vi "RT_Main.vi"() -> ()   [LabVIEW 2018]
uses:
  controls/Data To Save.ctl
  controls/Control RT Code.ctl
  controls/Trial Config Settings.ctl
  <vilib>/Platform/TimedLoop/XDataNode/timing_clust.ctl
  <vilib>/Platform/TimedLoop/XDataNode/nitl_modes.ctl
  <vilib>/Platform/TimedLoop/XDataNode/wakeup.ctl
  controls/Rig Config Settings.ctl
  <vilib>/FPGAPlugInAG/cRIO-9045/niLvFpga_Open_cRIO-9045.vi
  <vilib>/rvi/interface/common/dynamic/niFpgaDynamicAddResources.vi
  <vilib>/FPGAPlugInAG/Dynamic/niLvFpga_Run_Dynamic.vi
  Globals/Global - Configuration Options.vi
  <vilib>/FPGAPlugInAG/Dynamic/niLvFpga_Close_Dynamic.vi
  <vilib>/Platform/TimedLoop/XDataNode/XDataNode.xnode
  <vilib>/rvi/interface/nirviOpenFPGA/nirviOpenFPGA.xnode
  FPGA Bitfiles/UIUCWhiskerProje_FPGATarget_FPGABuild_ja8qmgOJlMY.lvbitx
  FPGA_Main.vi
  <vilib>/rvi/interface/nirviMethod/nirviMethod.xnode
  <vilib>/rvi/interface/nirviCloseFPGA/nirviCloseFPGA.xnode
  <vilib>/Platform/TimedLoop/XDataNode/XDNodeRunTimeDep.lvlib
  <vilib>/NI_Real-Time Target Support.lvlib
  <vilib>/FPGAPlugInAG/Dynamic/niLvFpga_Abort_Dynamic.vi
  <vilib>/FPGAPlugInAG/Dynamic/niLvFpga_Reset_Dynamic.vi
panel:
  out "Group Size for Randomization":i32
  out "Trial Running Graph Flag":bool
  out "Trial#":i16
  out "Super Trial Group on Test":string[](array[string])
  in  "Inter Group Counter":dbl
  out "Super Trial Groups":i32
  out "Super Trial Groups":string[][](array[string])
  out "Start Test":bool
  out "Test Trial Plot Color Array":u32[](array[numeric])
  out "Test Trial Array":string[](array[string])
  out "Numeric":i32
  out "Flag - Lat Dist History":bool
  out "Lateral Trial History":dbl[][](array[numeric])
  out "# water at start of new trial":i32
  out "Array":T1[](array[typedef])
  out "RT Loop Finished Late?":bool
  out "cur_trial_distance":dbl
  out "Analog Inputs":sgl[](array[numeric])
  out "Analog Outputs":sgl[](array[numeric])
  out "DIO":bool[](array[boolean])
  out "Trial In Progress":T2
  out "Time into Trial":dbl
  out "Trial Config Index":i32
  in  "Inter-Trial Interval":bool
  out "Test Trial In Progress":string
  out "Trial Tracker":string[][](table)=[["Test Reward.dat", "9", "8"], ["Test NO Reward.dat", "8", "0"]]
  out "Array of Trial File Names":string[](array[string])
  in  "Test Trial Index":i32
  out "Array of Trials":T2[](array[typedef])
  out "Timeout Timer":dbl format="%.3f"
  out "Timeout?":bool
  out "Timeout SP":dbl caption="Timeout" format="%.1f"
  out "Trial Fraction":dbl format="%.2f"
  in  "Command RT Code":T1
  out "# elements":u32
  out "Flash Drive Directory":path=path "u:/"
  out "# of CPUs":u32
  out "Error Out":errorcluster
  in  "Error In":errorcluster
  out "Data To Save":T3 {"Seconds Into Trial(s)" format="%#.10g"}
  out "Trial Running":bool
  out "Loop Rate for High Priority Acq Loop":u32
  out "cRIO System Time":string
  out "cRIO System Date":string
  out "cRIO CPU1 Usage":dbl format="%.2f"
  out "cRIO CPU2 Usage":dbl format="%.2f"
  # "Inputs and Outputs"
  # "aClck_DI"
  # "frame_clock_DO"
  # "whisker_video_ctrl_DO"
  # "lick_signal_DO"
  # "water_valve_ctrl_DO"
  # "laser_ctrl"
  # "left_texture_ctrl_DO"
  # "right_texture_ctrl_DO"
  # "trial_ephys_ctrl_DO"
  # "trial_iti_ctrl_DO"
  # "trial_on_ctrl_DO"
  # "ephys_clock_DO"
  # "Timeout"
  # "cm"
  # "secs"
  # "secs"
  # "secs"
  # "msec"
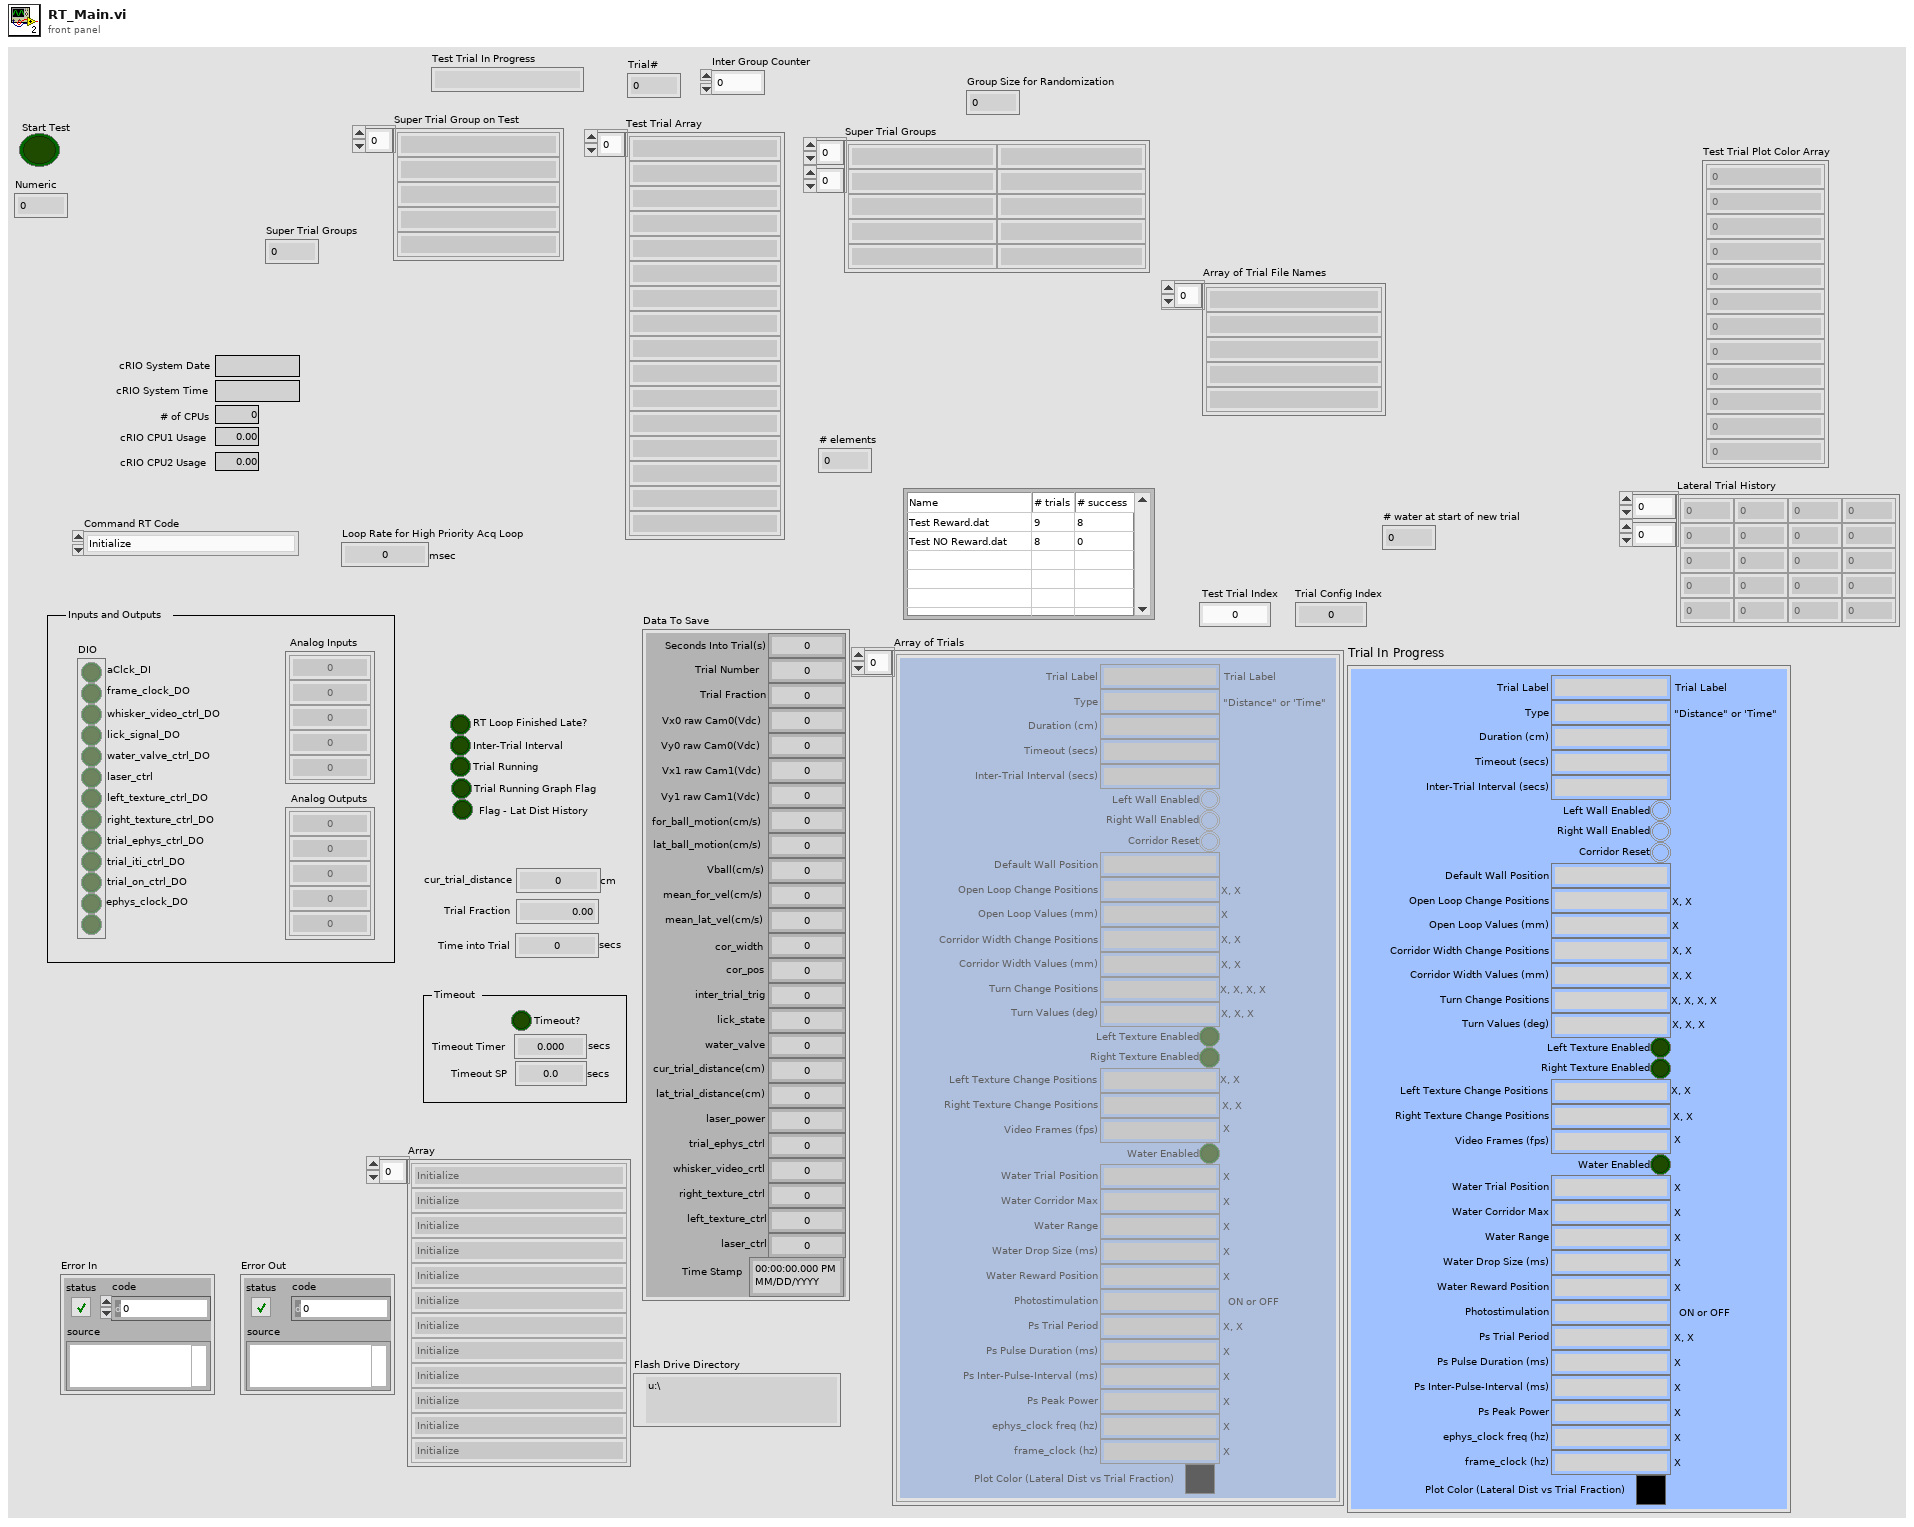
[diagram p1: front panel]
types:
  T1 = typedef "Control RT Code.ctl" = enum16{"Initialize", "Start New Test", "Stop Trial", "Start New Trial", "Load Trial Config Settings", "Load Rig Config Settings", "Determine Which Trial to Run", "Download All Trials to RT System", "Create New Folder", "Create New Data File", "Inter-Trial Interval Delay", "Initialize Trial Tracker", "Update Water Tracker", "Update Trial Tracker", "Exit"}
  T2 = typedef "Trial Config Settings.ctl" = cluster{"Trial Label":string, "Type":string, "Timeout (secs)":string, "Inter-Trial Interval (secs)":string, "Left Wall Enabled":bool, "Right Wall Enabled":bool, "Corridor Reset":bool, "Default Wall Position":string, "Open Loop Change Positions":string, "Open Loop Values (mm)":string, "Corridor Width Change Positions":string, "Corridor Width Values (mm) ":string, "Turn Change Positions":string, "Turn Values (deg)":string, "Left Texture Change Positions":string, "Right Texture Change Positions":string, "Video Frames (fps)":string, "Water Enabled":bool, "Water Trial Position":string, "Photostimulation":string, "Water Corridor Max":string, "Water Range":string, "Water Drop Size (ms)":string, "Water Reward Position":string, "Duration (cm)":string, "Left Texture Enabled":bool, "Right Texture Enabled":bool, "Ps Trial Period":string, "Ps Inter-Pulse-Interval (ms)":string, "Ps Peak Power":string, "Ps Pulse Duration (ms)":string, "ephys_clock freq (hz)":string, "frame_clock (hz)":string, "Plot Color (Lateral Dist vs Trial Fraction)":u32}
  T3 = typedef "Data To Save.ctl" = cluster{"Vx0 raw Cam0(Vdc)":sgl, "Vy0 raw Cam0(Vdc)":sgl, "Vx1 raw Cam1(Vdc)":sgl, "Vy1 raw Cam1(Vdc)":sgl, "Seconds Into Trial(s)":dbl, "cor_width":sgl, "cor_pos":sgl, "for_ball_motion(cm/s)":sgl, "lat_ball_motion(cm/s)":sgl, "Vball(cm/s)":sgl, "mean_for_vel(cm/s)":sgl, "mean_lat_vel(cm/s)":sgl, "Trial Fraction":dbl, "Trial Number":i16, "inter_trial_trig":i16, "lick_state":i16, "water_valve":i16, "cur_trial_distance(cm)":dbl, "lat_trial_distance(cm)":dbl, "laser_power":dbl, "trial_ephys_ctrl":i16, "whisker_video_crtl":i16, "right_texture_ctrl":i16, "left_texture_ctrl":i16, "laser_ctrl":i16, "Time Stamp":timestamp}
  T4 = cluster{"read mode":enum16{"polling", "blocking"}, "write mode":enum16{"polling", "blocking"}}
  T5 = enum16{"Create Folder", "Save", "Create New Data File"}
  T6 = typedef "XDNodeRunTimeDep.lvlib/timing_clust.ctl" = cluster{"Expected End [f-1]":u64, "Actual End [f-1]":u64, "Finished Late? [f-1]":bool, "Expected End [i-1]":u64, "Actual End [i-1]":u64, "Finished Late? [i-1]":bool, "Expected Start [i]":u64, "Actual Start [i]":u64, "Expected Start [f]":u64, "Actual Start [f]":u64, "Source Name":string, "Structure Name":string, "Period":i64, "Deadline":i64, "Offset":i64, "Start":i64, "Priority":i32, "Timeout":i32, "Mode":T7, "Wakeup Reason":T8, "Error":errorcluster, "Source Type":string, "Secondary Source Type":string, "Global End Time":u64, "Global Start Time":u64, "Frame Duration":u64, "Iteration Duration":u64, "Assigned CPU":i32, "I/O Scan Engine Mode":u32}
  T7 = typedef "XDNodeRunTimeDep.lvlib/nitl_modes.ctl" = enum32{"No Change", "Process missed periods, maintain original phase", "Discard missed periods, maintain original phase", "Process missed periods, ignore original phase", "Discard missed periods, ignore original phase"}
  T8 = typedef "XDNodeRunTimeDep.lvlib/wakeup.ctl" = enum32{"Normal", "Aborted", "Asynchronous wakeup", "Timing source error", "Timed loop error", "Timeout"}
  T9 = typedef "Rig Config Settings.ctl" = cluster{"Rig Name":string, "Rig Room":string, "Base Directory":string, "Computer IP Address":string, "Globals Name":string, "Treatmill Str":string, "cRIO Test Data Dir":path, "ai":string, "ao":string, "dio":string, "A_calib_str_row1":string, "A_calib_str_row2":string, "A_calib_str_row3":string, "Zero_V_str":string, "step_V":string, "Sample Freq":string, "ai_threshold":string, "run_speed_thresh":string, "speed_time_length":string, "wall ball gain":string, "max wall pos":string, "max cor width":string, "Trial Config Directory":path, "Randomize Trials?":bool}
  T10 = typedef "NI_Real-Time Target Support.lvlib/RT CPU Load.ctl" = cluster{"Total (%)":dbl, "Time Critical (%)":dbl, "Timed Structures (%)":dbl, "High (%)":dbl, "Above Normal (%)":dbl, "Normal (%)":dbl, "Background (%)":dbl, "Idle (%)":dbl, "ISR (%)":dbl}
  T11 = cluster{"Frequency (periods/tick)":fxp<+,32,0>, "Phase offset (periods)":fxp<+,32,0>, "Scale factor":fxp<+/-,16,1>, "Amplitude offset":fxp<+/-,16,16>, "duty cycle (periods)":fxp<+,32,0>}
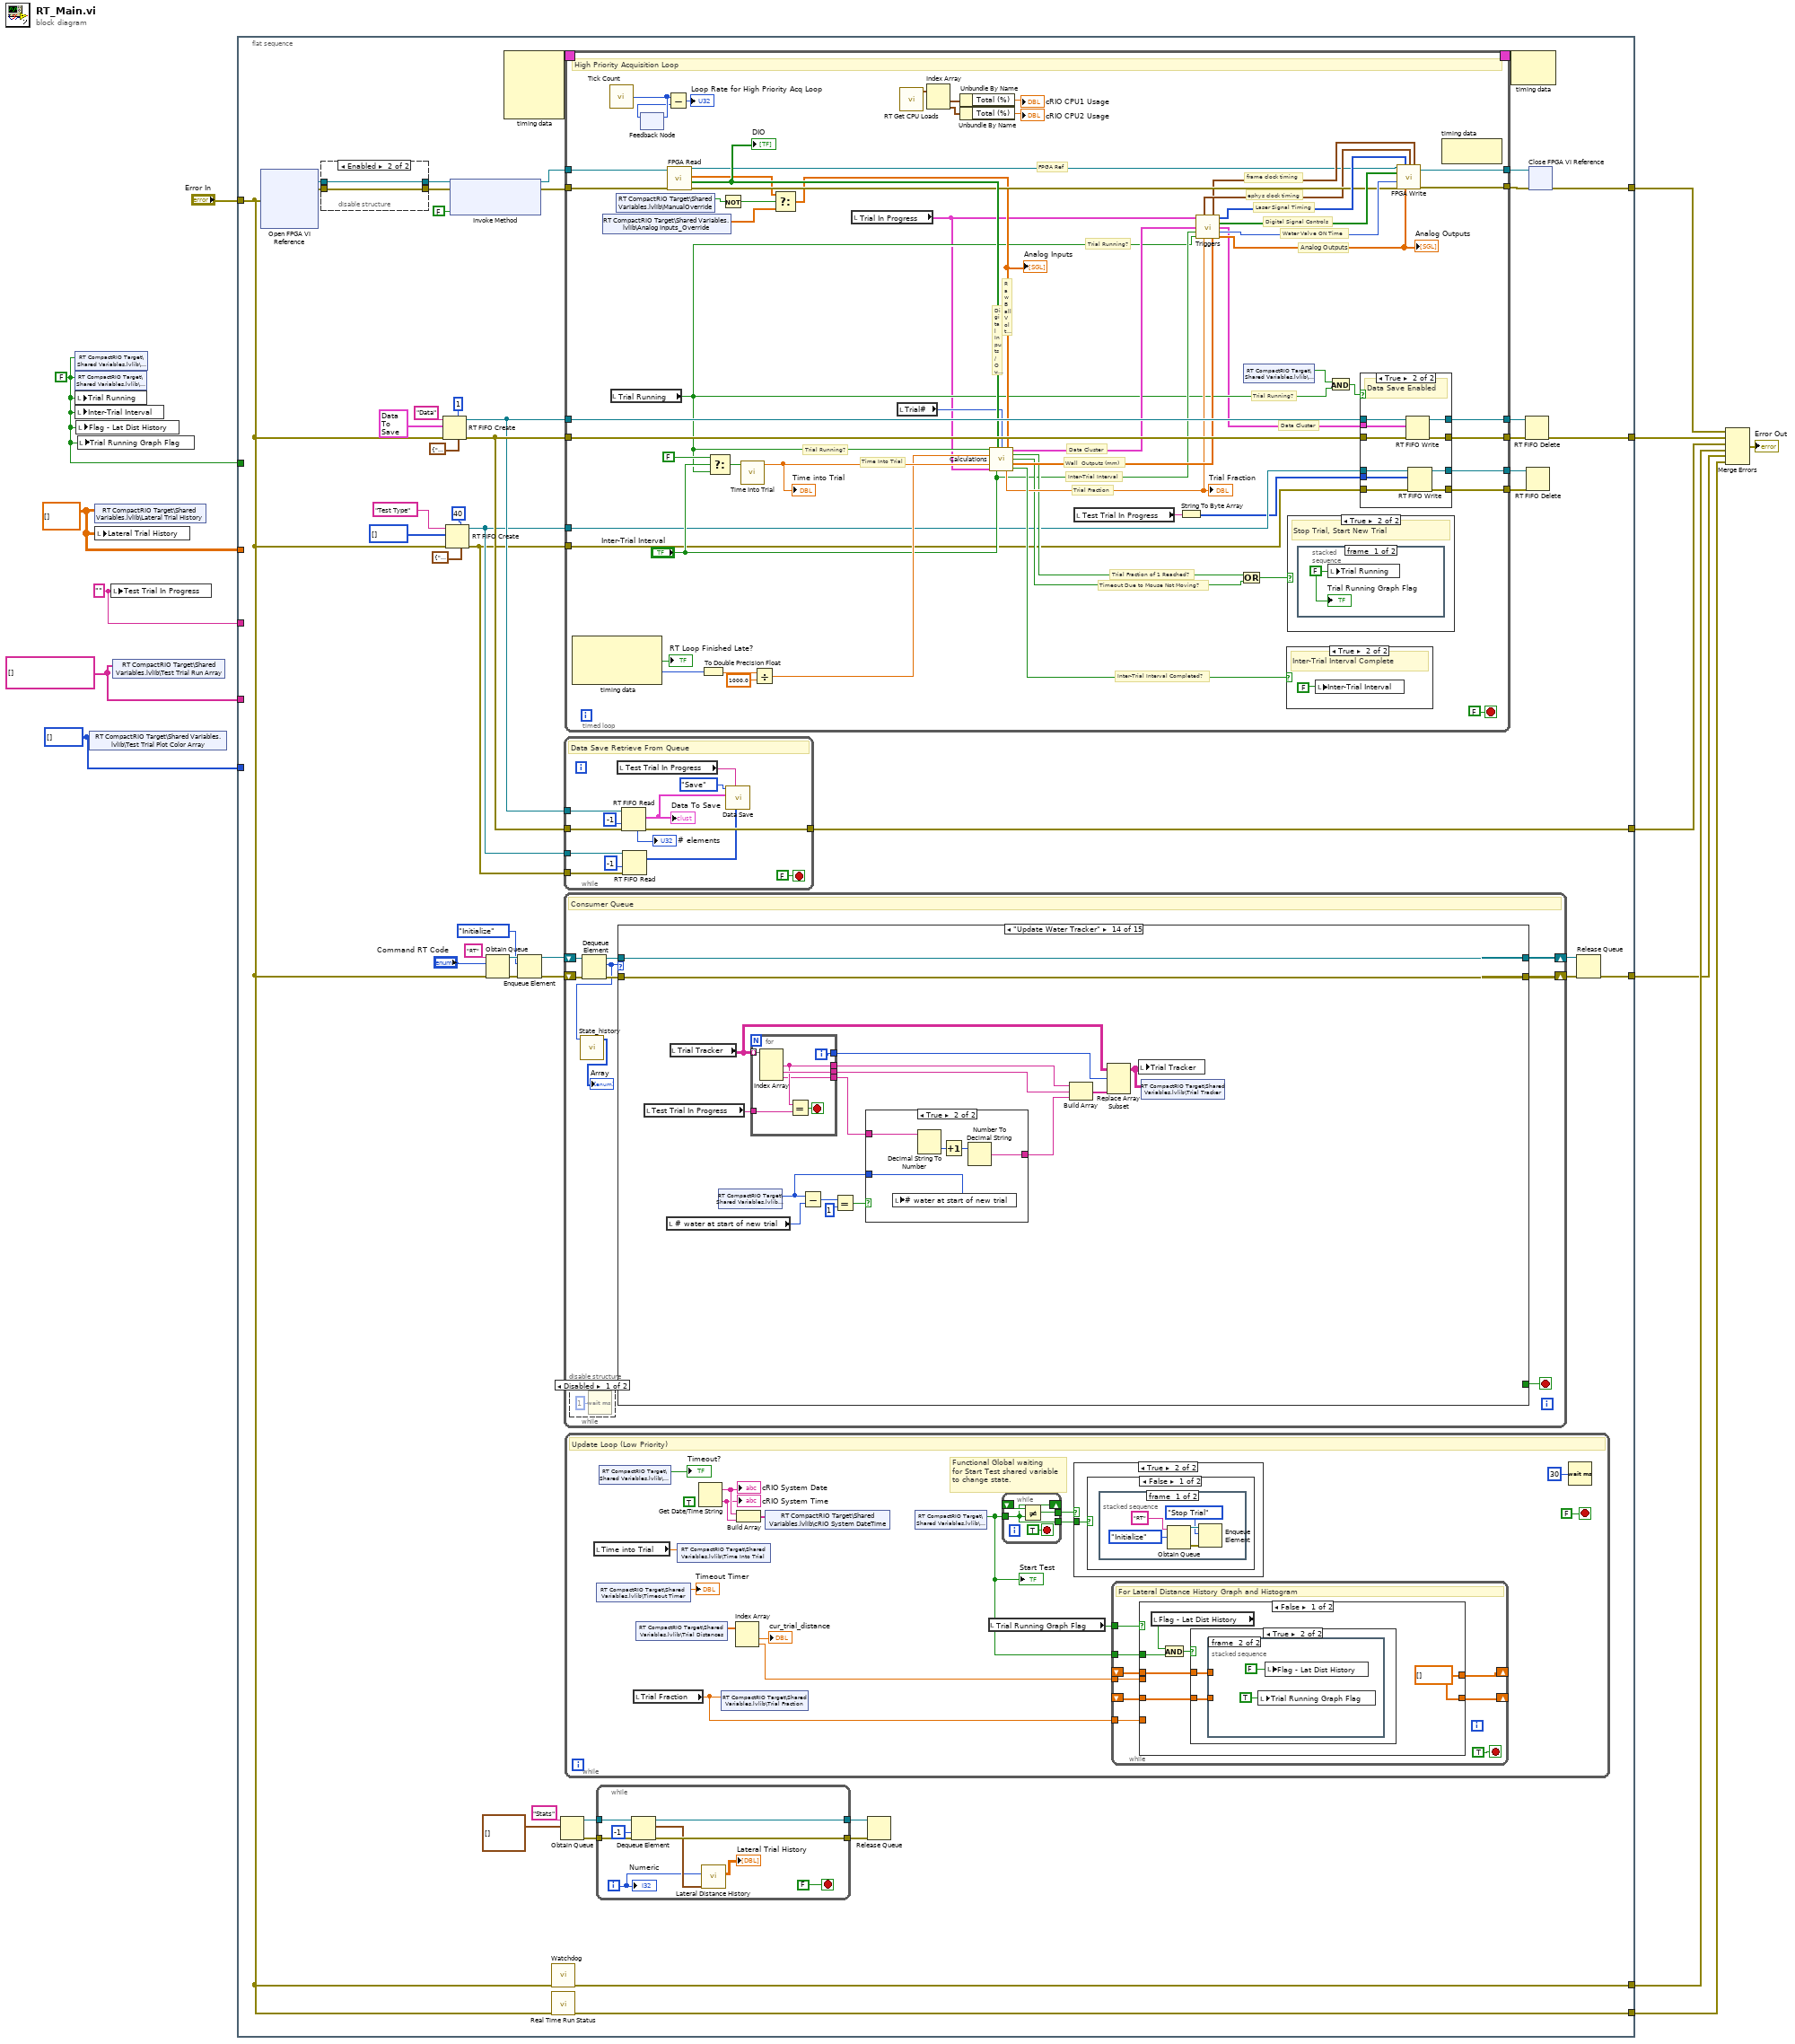
[diagram p0: block diagram]
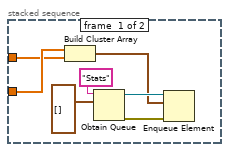
[diagram p3: hidden frame]
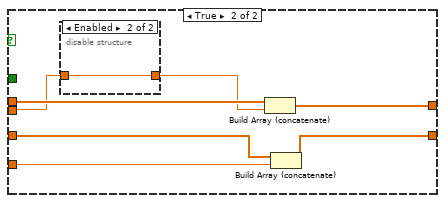
[diagram p4: hidden frame]
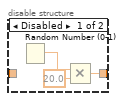
[diagram p5: hidden frame]
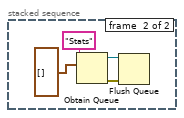
[diagram p7: hidden frame]
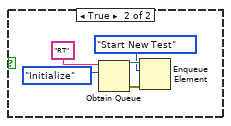
[diagram p8: hidden frame]
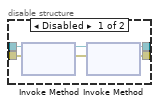
[diagram p9: hidden frame]
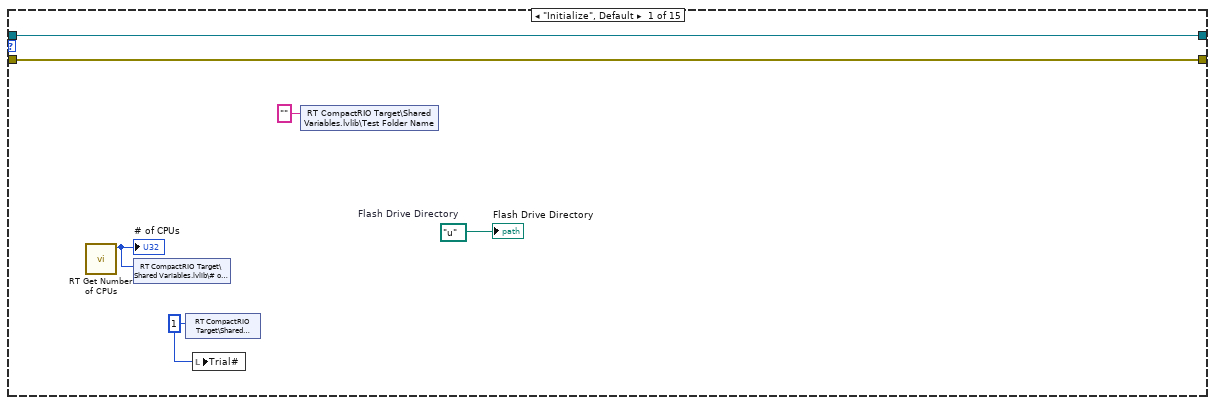
[diagram p11: hidden frame]
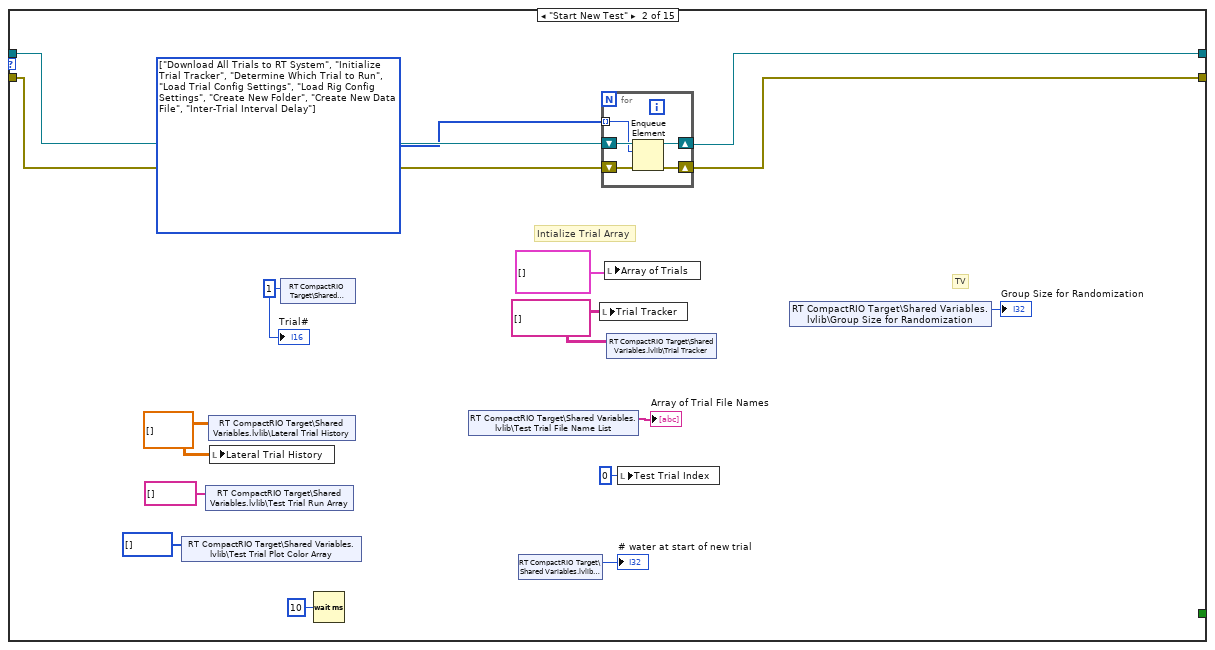
[diagram p12: hidden frame]
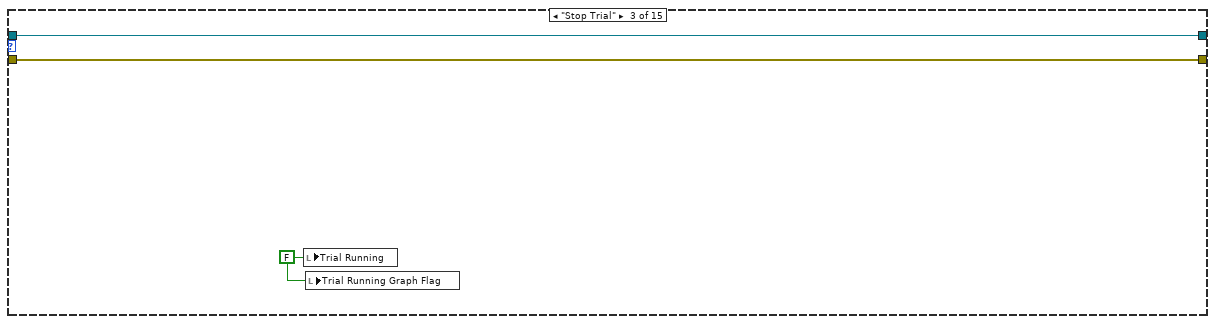
[diagram p13: hidden frame]
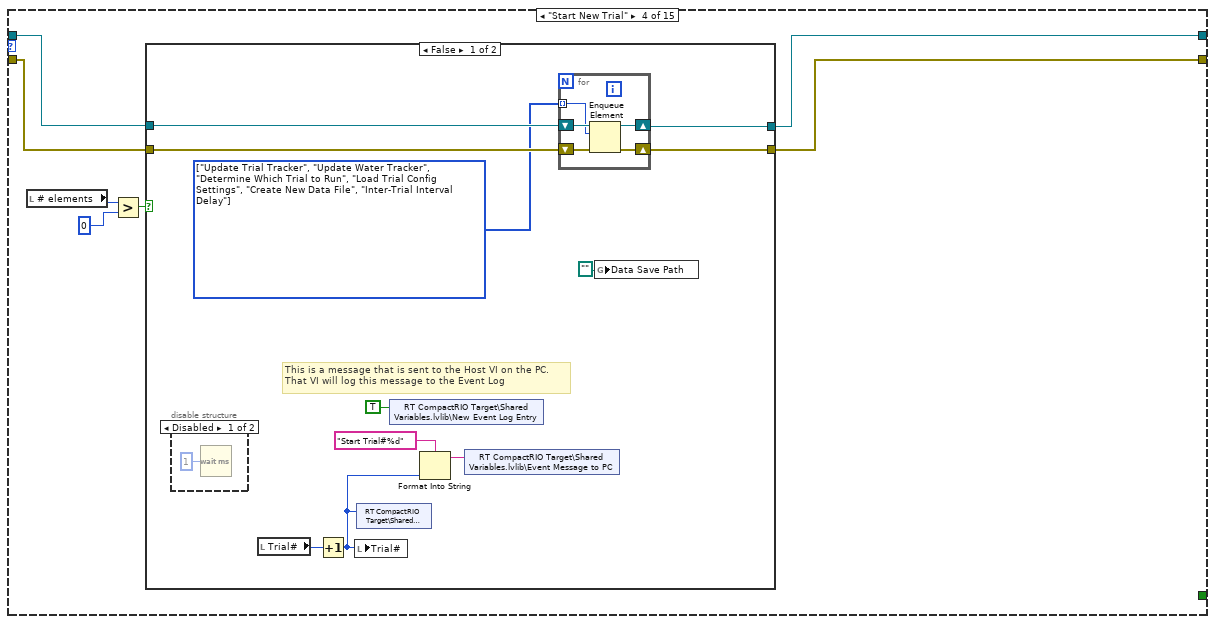
[diagram p14: hidden frame]
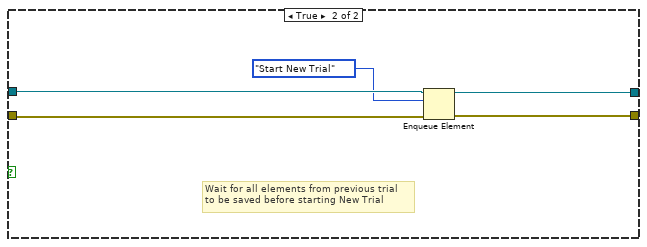
[diagram p16: hidden frame]
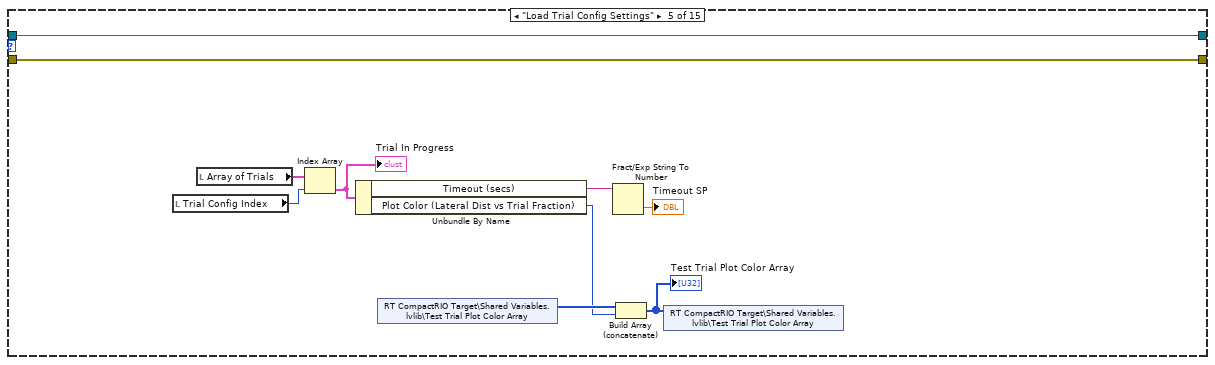
[diagram p17: hidden frame]
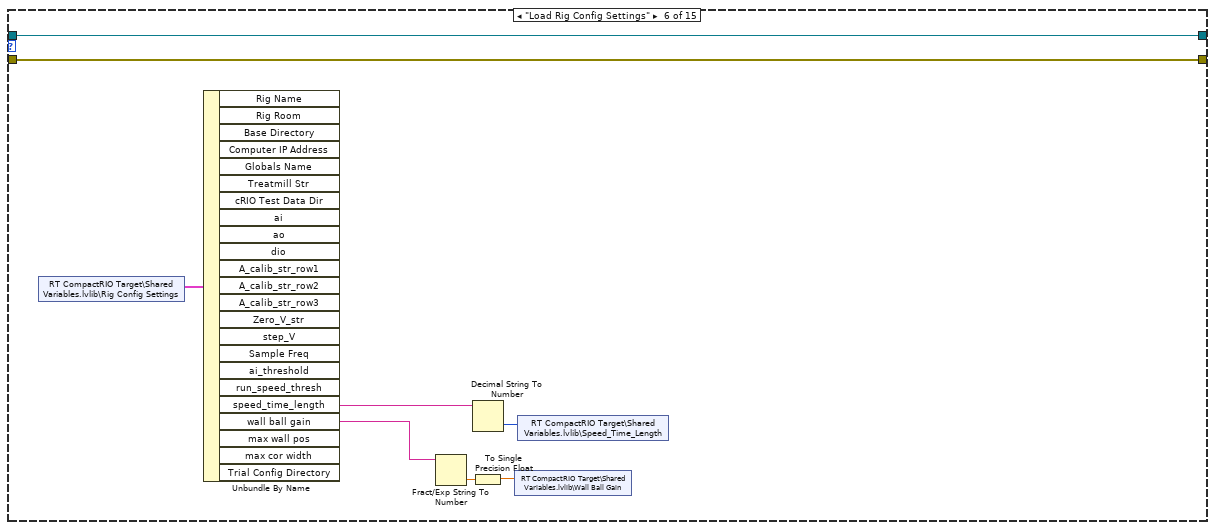
[diagram p18: hidden frame]
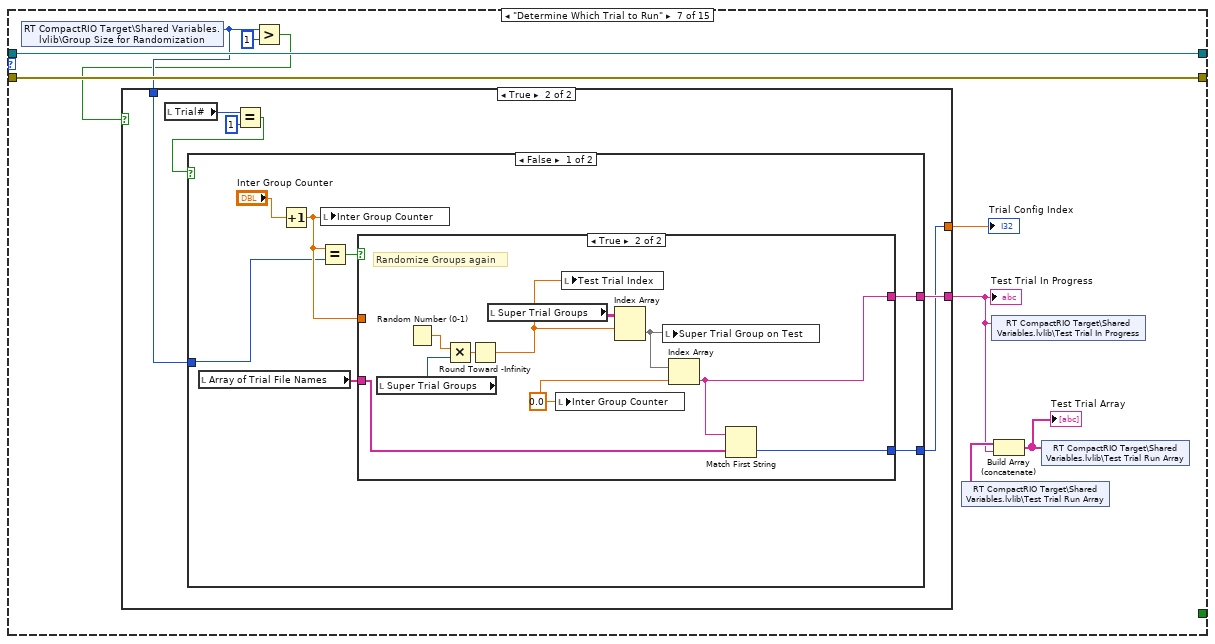
[diagram p19: hidden frame]
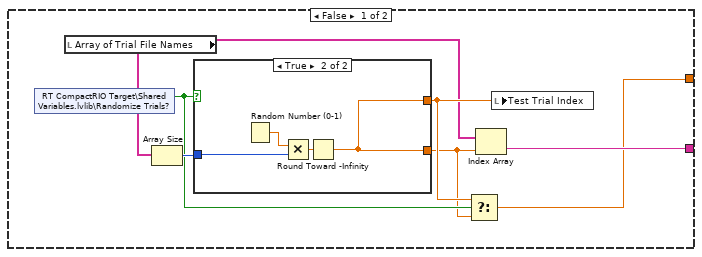
[diagram p20: hidden frame]
diagram:
  w2 = u32[] [] ("Test Trial Plot Color Array")
  w3 = string[] [] ("Test Trial Run Array")
  w4 = "" ("Test Trial In Progress")
  w5 = dbl[][] [] ("Histogram Data")
  w1 = FALSE ("Start Test for FPGA")
  n1 = shared-variable "RT CompactRIO Target\\Shared Variables.lvlib\\Timeout?"(w1) -> ()  [unwired: 1 in, 1 out]
  n2 = shared-variable "RT CompactRIO Target\\Shared Variables.lvlib\\Start Test"(w1) -> ()  [unwired: 1 in, 1 out]
  n3 = local write "Trial Running"(w1) -> ()
  n4 = local write "Inter-Trial Interval"(w1) -> ()
  n5 = local write "Flag - Lat Dist History"(w1) -> ()
  n6 = local write "Trial Running Graph Flag"(w1) -> ()
  n7 = shared-variable "RT CompactRIO Target\\Shared Variables.lvlib\\Test Trial Plot Color Array"(w2) -> ()  [unwired: 1 in, 1 out]
  n8 = shared-variable "RT CompactRIO Target\\Shared Variables.lvlib\\Lateral Trial History"(w5) -> ()  [unwired: 1 in, 1 out]
  n9 = local write "Lateral Trial History"(w5) -> ()
  n10 = local write "Test Trial In Progress"(w4) -> ()
  n11 = shared-variable "RT CompactRIO Target\\Shared Variables.lvlib\\Test Trial Run Array"(w3) -> ()  [unwired: 1 in, 1 out]
  n12 = flat-sequence {
    tunnel: [w54] -> w13
    tunnel: [w50] -> w12
    tunnel: [w44] -> w11
    tunnel: [w53] -> w10
    tunnel: [w47] -> w8
    tunnel: [w31] -> w7
    tunnel: "Error In" -> [w18]
    tunnel: w1 -> [_]
    tunnel: w5 -> [_]
    tunnel: w4 -> [_]
    tunnel: w3 -> [_]
    tunnel: w2 -> [_]
    frame #0 {
      n13 = xnode "Open FPGA VI Reference"("error in"=w18) -> ("FPGA VI Reference Out"=w48:refnum<k20>, "error out"=w57:errorcluster)  [unwired: 1 in]
      n14 = disable-structure shown="Enabled" {
        disable-tunnel: [w162 w164] -> w58
        disable-tunnel: w48 -> [w160 w164]
        disable-tunnel: w57 -> [w159 w163]
        disable-tunnel: [w157 w163] -> w56
        frame Disabled {
          n15 = xnode "Invoke Method"("FPGA VI Reference In"=w160, "error in"=w159) -> ("FPGA VI Reference Out"=w161:refnum<k20>, "error out"=w158:errorcluster)
          n16 = xnode "Invoke Method"("FPGA VI Reference In"=w161, "error in"=w158) -> ("FPGA VI Reference Out"=w162:refnum<k20>, "error out"=w157:errorcluster)
        }
        frame Enabled {
        }
      }
      n17 = RT FIFO Create(0:"Data" ("name (unnamed)"), 1:T3 {"Vx0 raw Cam0(Vdc)"=0.0, "Vy0 raw Cam0(Vdc)"=0.0, "Vx1 raw Cam1(Vdc)"=0.0, "Vy1 raw Cam1(Vdc)"=0.0, "Seconds Into Trial(s)"=0.0, "cor_width"=0.0, "cor_pos"=0.0, "for_ball_motion(cm/s)"=0.0, "lat_ball_motion(cm/s)"=0.0, "Vball(cm/s)"=0.0, "mean_for_vel(cm/s)"=0.0, "mean_lat_vel(cm/s)"=0.0, "Trial Fraction"=0.0, "Trial Number"=0, "inter_trial_trig"=0, "lick_state"=0, "water_valve"=0, "cur_trial_distance(cm)"=0.0, "lat_trial_distance(cm)"=0.0, "laser_power"=0.0, "trial_ephys_ctrl"=0, "whisker_video_crtl"=0, "right_texture_ctrl"=0, "left_texture_ctrl"=0, "laser_ctrl"=0, "Time Stamp"=timestamp(0 s since 1904-01-01)} ("Data Cluster OUT"), 3:w18, 6:u32 1 ("elements in array (1)"), 7:T4 {"read mode"=enum."blocking", "write mode"=enum."blocking"} ("r/w modes (polling,polling)")) -> (8:w45:refnum<k33>, 11:w46:errorcluster)  [unwired: 3 in, 1 out]
      n18 = RT FIFO Create(0:"Test Type" ("name (unnamed)"), 1:u8[] [] ("Trial Type"), 3:w18, 6:u32 40 ("elements in array (1)"), 7:T4 {"read mode"=enum."blocking", "write mode"=enum."blocking"} ("r/w modes (polling,polling)")) -> (8:w17:refnum<k33>, 11:w15:errorcluster)  [unwired: 3 in, 1 out]
      n19 = xnode "Invoke Method"("FPGA VI Reference In"=w58, "error in"=w56, "Wait Until Done (F)"=FALSE) -> ("FPGA VI Reference Out"=w49:refnum<k20>, "error out"=w59:errorcluster)
      n20 = Obtain Queue(name (unnamed)="RT", element data type="Command RT Code", error in (no error)=w18) -> (queue out=w40:refnum<queue>, error out=w41:errorcluster)  [unwired: 2 in, 1 out]
      n21 = node-c288() -> (w62:T6)  [unwired: 4 in]
      n22 = Enqueue Element(queue=w40, element=Control_RT_Code."Initialize", error in (no error)=w41) -> (queue out=w38:refnum<queue>, error out=w37:errorcluster)  [unwired: 1 in, 1 out]
      n23 = call "Watchdog.vi"("Error IN"=w18) -> ("Error Out"=w53:errorcluster)  [unwired: 10 in]
      n24 = call "Real Time Run Status.vi"("Error IN"=w18) -> ("Error OUT"=w47:errorcluster)  [unwired: 9 in, 1 out]
      n25 = Obtain Queue(name (unnamed)="Stats", element data type=cluster{"Numeric":dbl, "Numeric":dbl}[] [] ("array of clusters")) -> (queue out=w26:refnum<queue>, error out=w25:errorcluster)  [unwired: 3 in, 1 out]
      n26 = while {
        tunnel: [w156] -> w44
        tunnel: w46 -> [w155]
        tunnel: w45 -> [w154]
        tunnel: w15 -> [w146]
        tunnel: w17 -> [w145]
        stop <- FALSE stop-if-true
        # "Data Save Retrieve From Queue"
        n27 = local read "Test Trial In Progress"() -> (w149:string)
        n28 = RT FIFO Read(0:w154, 2:-1 ("timeout in ms (0)"), 3:w155) -> (7:→"# elements":u32, 9:w148:T3, 11:w156:errorcluster)  [unwired: 1 in, 2 out]
        "Data To Save" <- w148
        n29 = RT FIFO Read(0:w145, 2:-1 ("timeout in ms (0)"), 3:w146) -> (9:w144:u8[])  [unwired: 1 in, 4 out]
        n30 = call "Data Save.vi"("Test Type"=w144, "Test Trial In Progress"=w149, "Data Cluster"=w148, "Task"=T5."Save") -> ()  [unwired: 6 in, 2 out]
      }
      n31 = while {
        shift-right: [w169] -> w34
        shift-left: w38 -> [w173]
        shift-right: [w168] -> w33
        shift-left: w37 -> [w172]
        stop <- w167 stop-if-true
        # "Consumer Queue"
        n32 = disable-structure shown="Disabled" {
          frame Disabled {
            n33 = Wait (ms)(milliseconds to wait=u32 1) -> ()  [unwired: 1 out]
          }
          frame Enabled {
          }
        }
        n34 = Dequeue Element(queue=w173, error in (no error)=w172) -> (queue out=w171:refnum<queue>, element=w166:T1, error out=w170:errorcluster)  [unwired: 1 in, 1 out]
        n35 = call "State_history.vi"("element"=w166) -> ("Array"=→"Array":T1[])  [unwired: 10 in]
        n36 = case shown="\"Update Water Tracker\"" w166 {
          tunnel: w171 -> [w178 w196 w204 w211 w243 w251 w260 w327 w331 w341 w368 w375 w399 w422 w438]
          tunnel: w170 -> [w177 w193 w203 w208 w238 w250 w259 w326 w330 w340 w367 w374 w398 w421 w437]
          tunnel: [w178 w195 w204 w210 w243 w251 w260 w327 w331 w341 w368 w375 w399 w422 w438] -> w169
          tunnel: [w177 w194 w203 w209 w238 w250 w259 w326 w329 w339 w367 w374 w398 w421 w437] -> w168
          tunnel: [_ _ _ _ _ _ _ _ _ _ _ _ _ _ TRUE] -> w167
          frame "Initialize", Default {
            w175 = 1 ("Trial#")
            w179 = path "u:/"  # Flash Drive Directory
            n37 = call <vilib>:"RT Get Number of CPUs.vi"() -> ("# of CPUs"=w180:u32)  [unwired: 10 in, 1 out]
            "# of CPUs" <- w180
            n38 = shared-variable "RT CompactRIO Target\\Shared Variables.lvlib\\# of CPUs"(w180) -> ()  [unwired: 1 in, 1 out]
            n39 = shared-variable "RT CompactRIO Target\\Shared Variables.lvlib\\Trial#"(w175) -> ()  [unwired: 1 in, 1 out]
            n40 = local write "Trial#"(w175) -> ()
            n41 = shared-variable "RT CompactRIO Target\\Shared Variables.lvlib\\Test Folder Name"("" ("Test Folder Name")) -> ()  [unwired: 1 in, 1 out]
            "Flash Drive Directory" <- w179
          }
          frame "Start New Test" {
            w183 = 1 ("Trial#")
            w187 = dbl[][] [] ("Histogram Data")
            w186 = string[][] [] ("Trial Tracker")
            w192 = T1[] [enum."Download All Trials to RT System", enum."Initialize Trial Tracker", enum."Determine Which Trial to Run", enum."Load Trial Config Settings", enum."Load Rig Config Settings", enum."Create New Folder", enum."Create New Data File", enum."Inter-Trial Interval Delay"] items=["Initialize", "Start New Test", "Stop Trial", "Start New Trial", "Load Trial Config Settings", "Load Rig Config Settings", "Determine Which Trial to Run", "Download All Trials to RT System", "Create New Folder", "Create New Data File", "Inter-Trial Interval Delay", "Initialize Trial Tracker", "Update Water Tracker", "Update Trial Tracker", "Exit"]
            # "TV"
            # "Intialize Trial Array"
            n42 = shared-variable "RT CompactRIO Target\\Shared Variables.lvlib\\Test Trial Plot Color Array"(u32[] [] ("Test Trial Plot Color Array")) -> ()  [unwired: 1 in, 1 out]
            n43 = shared-variable "RT CompactRIO Target\\Shared Variables.lvlib\\Test Trial Run Array"(string[] [] ("Test Trial Run Array")) -> ()  [unwired: 1 in, 1 out]
            n44 = shared-variable "RT CompactRIO Target\\Shared Variables.lvlib\\Lateral Trial History"(w187) -> ()  [unwired: 1 in, 1 out]
            n45 = local write "Lateral Trial History"(w187) -> ()
            n46 = shared-variable "RT CompactRIO Target\\Shared Variables.lvlib\\Trial#"(w183) -> ()  [unwired: 1 in, 1 out]
            n47 = Wait (ms)(milliseconds to wait=u32 10) -> ()  [unwired: 1 out]
            n48 = shared-variable "RT CompactRIO Target\\Shared Variables.lvlib\\Test Trial File Name List"() -> (→"Array of Trial File Names":string[])  [unwired: 1 in, 1 out]
            n49 = shared-variable "RT CompactRIO Target\\Shared Variables.lvlib\\# water"() -> (→"# water at start of new trial":i32)  [unwired: 1 in, 1 out]
            n50 = local write "Trial Tracker"(w186) -> ()
            n51 = for {
              shift-right: [w200] -> w195
              shift-left: w196 -> [w201]
              shift-right: [w198] -> w194
              shift-left: w193 -> [w199]
              tunnel: w192 -> [w197] mode=indexing
              n52 = Enqueue Element(queue=w201, element=w197, error in (no error)=w199) -> (queue out=w200:refnum<queue>, error out=w198:errorcluster)  [unwired: 1 in, 1 out]
            }
            n53 = local write "Array of Trials"(T2[] [] ("Array")) -> ()
            n54 = shared-variable "RT CompactRIO Target\\Shared Variables.lvlib\\Trial Tracker"(w186) -> ()  [unwired: 1 in, 1 out]
            n55 = local write "Test Trial Index"(0 ("Test Trial Index")) -> ()
            n56 = shared-variable "RT CompactRIO Target\\Shared Variables.lvlib\\Group Size for Randomization"() -> (→"Group Size for Randomization":i32)  [unwired: 1 in, 1 out]
            "Trial#" <- w183
          }
          frame "Stop Trial" {
            w202 = FALSE ("Trial Running")
            n57 = local write "Trial Running"(w202) -> ()
            n58 = local write "Trial Running Graph Flag"(w202) -> ()
          }
          frame "Start New Trial" {
            n59 = local read "# elements"() -> (w207:u32)
            n60 = Greater?(x=w207, y=u32 0) -> (0:w205:bool)
            n61 = case shown="False" w205 {
              tunnel: w211 -> [w222 w231]
              tunnel: [w221 w233] -> w210
              tunnel: [w220 w232] -> w209
              tunnel: w208 -> [w219 w230]
              frame False {
                w218 = T1[] [enum."Update Trial Tracker", enum."Update Water Tracker", enum."Determine Which Trial to Run", enum."Load Trial Config Settings", enum."Create New Data File", enum."Inter-Trial Interval Delay"] items=["Initialize", "Start New Test", "Stop Trial", "Start New Trial", "Load Trial Config Settings", "Load Rig Config Settings", "Determine Which Trial to Run", "Download All Trials to RT System", "Create New Folder", "Create New Data File", "Inter-Trial Interval Delay", "Initialize Trial Tracker", "Update Water Tracker", "Update Trial Tracker", "Exit"]
                # "This is a message that is sent to the Host VI on the PC.\nThat VI will log this message to the Event Log"
                n62 = disable-structure shown="Disabled" {
                  frame Disabled {
                    n63 = Wait (ms)(milliseconds to wait=u32 1) -> ()  [unwired: 1 out]
                  }
                  frame Enabled {
                  }
                }
                n64 = local read "Trial#"() -> (w213:i16)
                n65 = Increment(x=w213) -> (x+1=w212:i16)
                n66 = local write "Trial#"(w212) -> ()
                n67 = shared-variable "RT CompactRIO Target\\Shared Variables.lvlib\\Trial#"(w212) -> ()  [unwired: 1 in, 1 out]
                n68 = shared-variable "RT CompactRIO Target\\Shared Variables.lvlib\\New Event Log Entry"(TRUE ("New Event Log Entry")) -> ()  [unwired: 1 in, 1 out]
                n69 = Format Into String(format string="Start Trial#%d", w212) -> (resulting string=w214:string)  [unwired: 2 in, 1 out]
                n70 = shared-variable "RT CompactRIO Target\\Shared Variables.lvlib\\Event Message to PC"(w214) -> ()  [unwired: 1 in, 1 out]
                n71 = for {
                  shift-right: [w227] -> w221
                  shift-left: w222 -> [w228]
                  shift-right: [w225] -> w220
                  shift-left: w219 -> [w226]
                  tunnel: w218 -> [w224] mode=indexing
                  n72 = Enqueue Element(queue=w228, element=w224, error in (no error)=w226) -> (queue out=w227:refnum<queue>, error out=w225:errorcluster)  [unwired: 1 in, 1 out]
                }
                n73 = global write "Global - Configuration Options.vi" "Data Save Path"(path "") -> ()
              }
              frame True {
                # "Wait for all elements from previous trial\nto be saved before starting New Trial"
                n74 = Enqueue Element(queue=w231, element=Control_RT_Code."Start New Trial", error in (no error)=w230) -> (queue out=w233:refnum<queue>, error out=w232:errorcluster)  [unwired: 1 in, 1 out]
              }
            }
          }
          frame "Load Trial Config Settings" {
            n75 = local read "Trial Config Index"() -> (w237:i32)
            n76 = local read "Array of Trials"() -> (w240:T2[])
            n77 = Index Array(array=w240, index=w237) -> (element=w239:T2)
            "Trial In Progress" <- w239
            n78 = Unbundle By Name(w239) -> ("Timeout (secs)"=w241:string, "Plot Color (Lateral Dist vs Trial Fraction)"=w235:u32)
            n79 = shared-variable "RT CompactRIO Target\\Shared Variables.lvlib\\Test Trial Plot Color Array"() -> (w236:u32[])  [unwired: 1 in, 1 out]
            n80 = Fract/Exp String To Number(string=w241) -> (number=→"Timeout SP":dbl)  [unwired: 3 in, 1 out]
            n81 = Build Array (concatenate)(w236, w235) -> (w234:u32[])
            "Test Trial Plot Color Array" <- w234
            n82 = shared-variable "RT CompactRIO Target\\Shared Variables.lvlib\\Test Trial Plot Color Array"(w234) -> ()  [unwired: 1 in, 1 out]
          }
          frame "Load Rig Config Settings" {
            n83 = shared-variable "RT CompactRIO Target\\Shared Variables.lvlib\\Rig Config Settings"() -> (w249:T9)  [unwired: 1 in, 1 out]
            n84 = Unbundle By Name(w249) -> ("speed_time_length"=w248:string, "wall ball gain"=w246:string)  [unwired: 21 out]
            n85 = Fract/Exp String To Number(string=w246) -> (number=w245:dbl)  [unwired: 3 in, 1 out]
            n86 = Decimal String To Number(string=w248) -> (number=w247:i32)  [unwired: 2 in, 1 out]
            n87 = To Single Precision Float(number=w245) -> (single precision float=w244:sgl)
            n88 = shared-variable "RT CompactRIO Target\\Shared Variables.lvlib\\Wall Ball Gain"(w244) -> ()  [unwired: 1 in, 1 out]
            n89 = shared-variable "RT CompactRIO Target\\Shared Variables.lvlib\\Speed_Time_Length"(w247) -> ()  [unwired: 1 in, 1 out]
          }
          frame "Determine Which Trial to Run" {
            n90 = shared-variable "RT CompactRIO Target\\Shared Variables.lvlib\\Group Size for Randomization"() -> (w254:i32)  [unwired: 1 in, 1 out]
            n91 = Greater?(x=w254, y=1) -> (0:w253:bool)
            n92 = case shown="True" w253 {
              tunnel: [w262 w284] -> w256
              tunnel: w254 -> [_ w283]
              tunnel: [w261 w280] -> w252
              frame False {
                n93 = shared-variable "RT CompactRIO Target\\Shared Variables.lvlib\\Randomize Trials?"() -> (w264:bool)  [unwired: 1 in, 1 out]
                n94 = local read "Array of Trial File Names"() -> (w266:string[])
                n95 = Array Size(array=w266) -> (size(s)=w265:i32)
                n96 = case shown="True" w264 {
                  tunnel: [w270 w275] -> w263
                  tunnel: w265 -> [w272 w276]
                  tunnel: [w269 w275] -> w267
                  frame False {
                    n97 = Decrement(x=w272) -> (x-1=w271:i32)
                    n98 = Greater?(x="Test Trial Index", y=w271) -> (0:w274:bool)
                    n99 = Select(t=0, s=w274, f="Test Trial Index") -> (s? t:f=w270:i32)
                    n100 = Increment(x=w270) -> (x+1=w269:i32)
                  }
                  frame True {
                    n101 = Random Number (0-1)() -> (number: 0 to 1=w278:dbl)
                    n102 = Multiply(x=w278, y=w276) -> (x*y=w277:dbl)
                    n103 = Round Toward -Infinity(1:w277) -> (0:w275:dbl)
                  }
                }
                n104 = Select(t=w267, s=w264, f=w263) -> (s? t:f=w261:dbl)
                n105 = Index Array(array=w266, index=w263) -> (element=w262:string)
                n106 = local write "Test Trial Index"(w267) -> ()
              }
              frame True {
                n107 = local read "Trial#"() -> (w279:i16)
                n108 = Equal?(x=w279, y=1) -> (x = y?=w281:bool)
                n109 = case shown="False" w281 {
                  tunnel: [w287 w309] -> w284
                  tunnel: w283 -> [w286 w308]
                  tunnel: [w285 w307] -> w280
                  frame False {
                    n110 = local read "Array of Trial File Names"() -> (w291:string[])
                    n111 = Increment(x="Inter Group Counter") -> (x+1=w290:dbl)
                    n112 = Equal?(x=w290, y=w286) -> (x = y?=w289:bool)
                    n113 = local write "Inter Group Counter"(w290) -> ()
                    n114 = case shown="True" w289 {
                      tunnel: w290 -> [w295 _]
                      tunnel: w291 -> [w294 w299]
                      tunnel: [w293 w298] -> w287
                      tunnel: [w292 w297] -> w285
                      frame False {
                        n115 = local read "Super Trial Group on Test"() -> (w296:string[])
                        n116 = Index Array(array=w296, index=w295) -> (element=w293:string)
                        n117 = Match First String(2:w294, 3:w293) -> (0:w292:i32)  [unwired: 1 out]
                      }
                      frame True {
                        w301 = 0.0 ("Inter Group Counter")
                        # "Randomize Groups again"
                        n118 = local read "Super Trial Groups"() -> (w304:i32)
                        n119 = Random Number (0-1)() -> (number: 0 to 1=w306:dbl)
                        n120 = Multiply(x=w306, y=w304) -> (x*y=w305:dbl)
                        n121 = Round Toward -Infinity(1:w305) -> (0:w300:dbl)
                        n122 = local read "Super Trial Groups"() -> (w303:string[][])
                        n123 = local write "Inter Group Counter"(w301) -> ()
                        n124 = local write "Test Trial Index"(w300) -> ()
                        n125 = Index Array(array=w303, index (row)=w300) -> (element=w302:string[])  [unwired: 1 in]
                        n126 = local write "Super Trial Group on Test"(w302) -> ()
                        n127 = Index Array(array=w302, index=w301) -> (element=w298:string)
                        n128 = Match First String(2:w299, 3:w298) -> (0:w297:i32)  [unwired: 1 out]
                      }
                    }
                  }
                  frame True {
                    w317 = 0.0 ("Inter Group Counter")
                    n129 = local read "Array of Trial File Names"() -> (w319:string[])
                    n130 = Array Size(array=w319) -> (size(s)=w311:i32)
                    n131 = Divide(x=w311, y=w308) -> (x/y=w314:dbl)
                    "Super Trial Groups" <- w314
                    n132 = for {
                      N: w314 -> [_]
                      tunnel: w319 -> [w324]
                      tunnel: w308 -> [w322]
                      shift-right: [w320] -> _
                      shift-left: 0 -> [w323]
                      tunnel: [w321] -> w315 mode=indexing
                      n133 = Add(x=w323, y=w322) -> (x+y=w320:i32)
                      n134 = Array Subset(array=w324, index=w323, length=w322) -> (w321:string[])
                    }
                    "Super Trial Groups" <- w315
                    n135 = Random Number (0-1)() -> (number: 0 to 1=w313:dbl)
                    n136 = Multiply(x=w313, y=w314) -> (x*y=w312:dbl)
                    n137 = Round Toward -Infinity(1:w312) -> (0:w318:dbl)
                    n138 = Index Array(array=w315, index (row)=w318) -> (element=w316:string[])  [unwired: 1 in]
                    "Super Trial Group on Test" <- w316
                    n139 = local write "Test Trial Index"(w318) -> ()
                    n140 = local write "Inter Group Counter"(w317) -> ()
                    n141 = Index Array(array=w316, index=w317) -> (element=w309:string)
                    n142 = Match First String(2:w319, 3:w309) -> (0:w307:i32)  [unwired: 1 out]
                  }
                }
              }
            }
            "Test Trial In Progress" <- w256
            "Trial Config Index" <- w252
            n143 = shared-variable "RT CompactRIO Target\\Shared Variables.lvlib\\Test Trial Run Array"() -> (w258:string[])  [unwired: 1 in, 1 out]
            n144 = shared-variable "RT CompactRIO Target\\Shared Variables.lvlib\\Test Trial In Progress"(w256) -> ()  [unwired: 1 in, 1 out]
            n145 = Build Array (concatenate)(w258, w256) -> (w257:string[])
            "Test Trial Array" <- w257
            n146 = shared-variable "RT CompactRIO Target\\Shared Variables.lvlib\\Test Trial Run Array"(w257) -> ()  [unwired: 1 in, 1 out]
          }
          frame "Download All Trials to RT System" {
            n147 = shared-variable "RT CompactRIO Target\\Shared Variables.lvlib\\Trial Cluster Array"() -> (→"Array of Trials":T2[])  [unwired: 1 in, 1 out]
          }
          frame "Create New Folder" {
            n148 = shared-variable "RT CompactRIO Target\\Shared Variables.lvlib\\SaveData"() -> (w328:bool)  [unwired: 1 in, 1 out]
            n149 = case shown="True" w328 {
              tunnel: w330 -> [w332 w337]
              tunnel: [w332 w336] -> w329
              frame False {
              }
              frame True {
                # "This is a message that is sent to the Host VI on the PC.\nThat VI will log this message to the Event Log"
                n150 = shared-variable "RT CompactRIO Target\\Shared Variables.lvlib\\Event Message to PC"("Create Folder" ("Event Message to PC")) -> ()  [unwired: 1 in, 1 out]
                n151 = shared-variable "RT CompactRIO Target\\Shared Variables.lvlib\\New Event Log Entry"(TRUE ("New Event Log Entry")) -> ()  [unwired: 1 in, 1 out]
                n152 = call "Data Save.vi"("Error IN"=w337, "Task"=T5."Create Folder") -> ("Error OUT"=w336:errorcluster)  [unwired: 8 in, 1 out]
              }
            }
          }
          frame "Create New Data File" {
            n153 = shared-variable "RT CompactRIO Target\\Shared Variables.lvlib\\SaveData"() -> (w338:bool)  [unwired: 1 in, 1 out]
            n154 = case shown="True" w338 {
              tunnel: w340 -> [w342 w347]
              tunnel: [w342 w346] -> w339
              frame False {
              }
              frame True {
                # "TV"
                n155 = local read "Group Size for Randomization"() -> (w343:i32)
                n156 = Greater?(x=w343, y=1) -> (0:w344:bool)
                n157 = case shown="True" w344 {
                  tunnel: w347 -> [w350 w361]
                  tunnel: [w349 w360] -> w346
                  frame False {
                    # "TV"
                    # "This is not a group randomization test so create the data file as normal."
                    n158 = local read "Trial#"() -> (w348:i16)
                    n159 = call "Data Save.vi"("Error IN"=w350, "Trial#"=w348, "Task"=T5."Create New Data File") -> ("Error OUT"=w349:errorcluster)  [unwired: 7 in, 1 out]
                  }
                  frame True {
                    # "This is a group randomization test."
                    n160 = local read "Trial In Progress"() -> (w358:T2)
                    n161 = Unbundle By Name(w358) -> ("Inter-Trial Interval (secs)"=w359:string)
                    n162 = local read "Inter Group Counter"() -> (w357:dbl)
                    n163 = Equal?(x=w357, y=0.0) -> (x = y?=w355:bool)
                    n164 = Equal?(x=w359, y="0") -> (x = y?=w356:bool)
                    n165 = Compound Arithmetic op=AND(w356, w355) -> (w352:bool)
                    n166 = case shown="True" w352 {
                      tunnel: w361 -> [w362 w366]
                      tunnel: [w362 w365] -> w360
                      frame False {
                        # "Not the first test in the group so do not\nstart a new data file"
                      }
                      frame True {
                        # "First trial in the group so create a new data file"
                        n167 = local read "Trial#"() -> (w363:i16)
                        n168 = call "Data Save.vi"("Error IN"=w366, "Trial#"=w363, "Task"=T5."Create New Data File") -> ("Error OUT"=w365:errorcluster)  [unwired: 7 in, 1 out]
                      }
                    }
                  }
                }
              }
            }
          }
          frame "Inter-Trial Interval Delay" {
            n169 = flat-sequence {
              frame #0 {
                n170 = local write "Inter-Trial Interval"(TRUE ("Start Inter-Trial Delay?")) -> ()
              }
              frame #1 {
                n171 = Wait (ms)(milliseconds to wait=u32 3) -> ()  [unwired: 1 out]
              }
              frame #2 {
                w371 = TRUE ("Trial Running")
                "Trial Running" <- w371
                "Flag - Lat Dist History" <- w371
              }
            }
          }
          frame "Initialize Trial Tracker" {
            n172 = flat-sequence {
              tunnel: [w377] -> w373
              tunnel: [w376] -> w372
              tunnel: w373 -> [w380]
              tunnel: w372 -> [w379]
              frame #0 {
                w377 = string[][] [] ("Trial Tracker")
                n173 = local read "Array of Trial File Names"() -> (w376:string[])
                n174 = local write "Trial Tracker"(w377) -> ()
              }
              frame #1 {
                n175 = for {
                  shift-right: [w384] -> w378
                  shift-left: w380 -> [w386]
                  tunnel: w379 -> [w383] mode=indexing
                  i -> [w385]
                  w381 = "0" ("element")
                  n176 = Build Array(w383, w381, w381) -> (w382:string[])
                  n177 = Insert Into Array(array=w386, index (row)=w385, new element=w382) -> (w384:string[][])  [unwired: 1 in]
                }
                "Trial Tracker" <- w378
                n178 = shared-variable "RT CompactRIO Target\\Shared Variables.lvlib\\Trial Tracker"(w378) -> ()  [unwired: 1 in, 1 out]
              }
            }
          }
          frame "Update Trial Tracker" {
            n179 = local read "Test Trial In Progress"() -> (w389:string)
            n180 = local read "Trial Tracker"() -> (w390:string[][])
            n181 = for {
              tunnel: w390 -> [w406] mode=indexing
              tunnel: [w405] -> w397
              tunnel: w389 -> [w404]
              tunnel: [w402] -> w393
              tunnel: [w401] -> w394
              tunnel: [w400] -> w387
              i -> [w401]
              stop <- w403 stop-if-true
              n182 = Index Array(array=w406) -> (element #1=w402:string, element #2=w405:string, element #3=w400:string)  [unwired: 3 in]
              n183 = Equal?(x=w402, y=w404) -> (x = y?=w403:bool)
            }
            n184 = Decimal String To Number(string=w397) -> (number=w396:i32)  [unwired: 2 in, 1 out]
            n185 = Increment(x=w396) -> (x+1=w395:i32)
            n186 = Number To Decimal String(number=w395) -> (decimal integer string=w392:string)  [unwired: 1 in]
            n187 = Build Array(w393, w392, w387) -> (w391:string[])
            n188 = Replace Array Subset(array=w390, new element=w391, index (row)=w394) -> (w388:string[][])  [unwired: 1 in]
            n189 = local write "Trial Tracker"(w388) -> ()
            n190 = shared-variable "RT CompactRIO Target\\Shared Variables.lvlib\\Trial Tracker"(w388) -> ()  [unwired: 1 in, 1 out]
          }
          frame "Update Water Tracker" {
            n191 = local read "Test Trial In Progress"() -> (w416:string)
            n192 = local read "# water at start of new trial"() -> (w414:i32)
            n193 = local read "Trial Tracker"() -> (w417:string[][])
            n194 = shared-variable "RT CompactRIO Target\\Shared Variables.lvlib\\# water"() -> (w407:i32)  [unwired: 1 in, 1 out]
            n195 = for {
              tunnel: w417 -> [w435] mode=indexing
              tunnel: [w434] -> w408
              tunnel: w416 -> [w433]
              tunnel: [w431] -> w419
              tunnel: [w430] -> w420
              tunnel: [w429] -> w409
              i -> [w430]
              stop <- w432 stop-if-true
              n196 = Index Array(array=w435) -> (element #1=w431:string, element #2=w434:string, element #3=w429:string)  [unwired: 3 in]
              n197 = Equal?(x=w431, y=w433) -> (x = y?=w432:bool)
            }
            n198 = Subtract(x=w407, y=w414) -> (x-y=w413:i32)
            n199 = Equal?(x=w413, y=1) -> (x = y?=w411:bool)
            n200 = case shown="True" w411 {
              tunnel: [w423 w426] -> w410
              tunnel: w409 -> [w423 w425]
              tunnel: w407 -> [_ w424]
              frame False {
              }
              frame True {
                n201 = local write "# water at start of new trial"(w424) -> ()
                n202 = Decimal String To Number(string=w425) -> (number=w427:i32)  [unwired: 2 in, 1 out]
                n203 = Increment(x=w427) -> (x+1=w428:i32)
                n204 = Number To Decimal String(number=w428) -> (decimal integer string=w426:string)  [unwired: 1 in]
              }
            }
            n205 = Build Array(w419, w408, w410) -> (w418:string[])
            n206 = Replace Array Subset(array=w417, new element=w418, index (row)=w420) -> (w415:string[][])  [unwired: 1 in]
            n207 = local write "Trial Tracker"(w415) -> ()
            n208 = shared-variable "RT CompactRIO Target\\Shared Variables.lvlib\\Trial Tracker"(w415) -> ()  [unwired: 1 in, 1 out]
          }
          frame "Exit" {
          }
        }
      }
      n209 = timed-loop {
        timing: w62 -> [_]
        timing-out: [_] -> w61
        tunnel: w49 -> [w474]
        tunnel: w59 -> [w478]
        tunnel: [w475] -> w55
        tunnel: [w476] -> w60
        tunnel: w45 -> [w484]
        tunnel: w46 -> [w483]
        tunnel: [w485] -> w52
        tunnel: [w486] -> w51
        tunnel: w17 -> [w445]
        tunnel: [w442] -> w16
        tunnel: w15 -> [w441]
        tunnel: [w440] -> w14
        stop <- FALSE stop-if-true
        # "Data Cluster"
        # "Inter-Trial Interval Completed?"
        # "Timeout Due to Mouse Not Moving?"
        # "Trial Fraction of 1 Reached?"
        # "Wall  Outputs (mm)"
        # "ephys clock timing"
        # "frame clock timing"
        # "Digital Signal Controls"
        # "Laser Signal Timing"
        # "Water Valve ON Time"
        # "Analog Outputs"
        # "FPGA Ref"
        # "Digital Inputs/Outputs"
        # "Trial Running?"
        # "Inter-Trial Interval"
        # "Trial Fraction"
        # "Trial Running?"
        # "Data Cluster"
        # "Trial Running?"
        # "Raw Ball Voltages"
        # "Time Into Trial"
        # "High Priority Acquisition Loop"
        n210 = node-c288() -> (→"RT Loop Finished Late?":bool, w459:i64)  [unwired: 1 in, 1 out]
        n211 = shared-variable "RT CompactRIO Target\\Shared Variables.lvlib\\Analog Inputs_Override"() -> (w458:sgl[])  [unwired: 1 in, 1 out]
        n212 = call "Tick Count"() -> ("Tick Count(mSec)"=w497:u32)
        n213 = local read "Trial Running"() -> (w450:bool)
        n214 = shared-variable "RT CompactRIO Target\\Shared Variables.lvlib\\ManualOverride"() -> (w452:bool)  [unwired: 1 in, 1 out]
        n215 = feedback #1() -> (w496:u32)  [unwired: 1 in]
        n216 = feedback-in #1(w497) -> ()
        n217 = Subtract(x=w497, y=w496) -> (x-y=→"Loop Rate for High Priority Acq Loop":u32)
        n218 = call "FPGA Read.vi"("error in (no error)"=w478, "FPGA VI Reference IN"=w474) -> ("error out"=w477:errorcluster, "DIO OUT"=w482:bool[], "Raw Ball Voltages OUT"=w457:sgl[], "FPGA VI Reference OUT"=w468:refnum<k20>)  [unwired: 6 in]
        "DIO" <- w482
        n219 = To Double Precision Float(number=w459) -> (double precision float=w460:dbl)
        n220 = Select(t=FALSE, s="Inter-Trial Interval", f=w450) -> (s? t:f=w454:bool)
        n221 = Not(x=w452) -> (.not. x?=w451:bool)
        n222 = call "Time Into Trial.vi"("Trial In Progress IN"=w454) -> ("Time Into Trial (secs) OUT"=w479:dbl)  [unwired: 10 in]
        "Time into Trial" <- w479
        n223 = Divide(x=w460, y=1000.0) -> (x/y=w461:dbl)
        n224 = Select(t=w457, s=w451, f=w458) -> (s? t:f=w456:sgl[])
        "Analog Inputs" <- w456
        n225 = local read "Trial In Progress"() -> (w444:T2)
        n226 = local read "Trial#"() -> (w447:i16)
        n227 = call <vilib>:"RT Get CPU Loads.vi"() -> ("CPU loads"=w490:T10[])  [unwired: 10 in, 1 out]
        n228 = Index Array(array=w490) -> (element #1=w489:T10, element #2=w488:T10)  [unwired: 2 in]
        n229 = Unbundle By Name(w489) -> ("Total (%)"=→"cRIO CPU1 Usage":dbl)
        n230 = Unbundle By Name(w488) -> ("Total (%)"=→"cRIO CPU2 Usage":dbl)
        n231 = call "Calculations.vi"("Trial in Progress IN"=w450, "DIO"=w482, "Trial Number"=w447, "cam_vel_ai_vlt"=w456, "Sample Rate(s)"=w461, "Time Into Trial IN"=w479, "Trial In Progress IN"=w444, "Inter-Trial Interval IN"="Inter-Trial Interval") -> ("Data Cluster OUT"=w466:T3, "Trial Fraction of 1 Reached?"=w465:bool, "Timeout Due to Mouse Not Moving?"=w463:bool, "Wall MM Outputs"=w471:sgl[], "Trial Fraction OUT"=w469:dbl, "Inter-Trial Interval Complete?"=w470:bool)  [unwired: 2 in]
        "Trial Fraction" <- w469
        n232 = local read "Test Trial In Progress"() -> (w439:string)
        n233 = String To Byte Array(string=w439) -> (unsigned byte array=w443:u8[])
        n234 = call "Triggers.vi"(0:"Trial In Progress IN"=w444, "Data Cluster IN"=w466, "Inter-Trial Interval IN"="Inter-Trial Interval", 11:"Trial In Progress IN"=w450, "Trial Fraction IN"=w469, "Wall Inputs (mm)"=w471) -> ("ephys Clock Timing OUT"=w473:T11, "Frame Clock Timing OUT"=w472:T11, "Laser Signal Timing OUT"=w493:i16[], "Digital Controls OUT"=w487:bool[], "Data Cluster OUT"=w446:T3, "Water Valve ON Time OUT"=w494:i32, "Analog Outputs OUT"=w480:sgl[])  [unwired: 3 in]
        "Analog Outputs" <- w480
        n235 = Or(x=w465, y=w463) -> (x .or. y?=w464:bool)
        n236 = shared-variable "RT CompactRIO Target\\Shared Variables.lvlib\\SaveData"() -> (w448:bool)  [unwired: 1 in, 1 out]
        n237 = case shown="True" w470 {
          frame False {
            # "Inter-Trial Interval In Progress"
          }
          frame True {
            # "Inter-Trial Interval Complete"
            n238 = local write "Inter-Trial Interval"(FALSE ("Start Inter-Trial Delay?")) -> ()
          }
        }
        n239 = case shown="True" w464 {
          frame False {
          }
          frame True {
            # "Stop Trial, Start New Trial"
            n240 = stacked-sequence {
              frame #0 {
                w512 = FALSE ("Trial Running")
                n241 = local write "Trial Running"(w512) -> ()
                "Trial Running Graph Flag" <- w512
              }
              frame #1 {
                n242 = Obtain Queue(name (unnamed)="RT", element data type=Control_RT_Code."Initialize" ("Command RT Code")) -> (queue out=w516:refnum<queue>)  [unwired: 3 in, 2 out]
                n243 = Enqueue Element(queue=w516, element=Control_RT_Code."Start New Trial") -> ()  [unwired: 2 in, 3 out]
              }
            }
          }
        }
        n244 = And(x=w448, y=w450) -> (x .and. y?=w449:bool)
        n245 = case shown="True" w449 {
          tunnel: w446 -> [_ w507]
          tunnel: [w501 w511] -> w486
          tunnel: [w500 w510] -> w485
          tunnel: w484 -> [w501 w508]
          tunnel: w483 -> [w500 w509]
          tunnel: w445 -> [w499 w506]
          tunnel: w443 -> [_ w505]
          tunnel: [w499 w504] -> w442
          tunnel: w441 -> [w498 w503]
          tunnel: [w498 w502] -> w440
          frame False {
            # "Data Save Disabled"
          }
          frame True {
            # "Data Save Enabled"
            n246 = RT FIFO Write(0:w508, 1:w507, 3:w509) -> (8:w511:refnum<k33>, 11:w510:errorcluster)  [unwired: 2 in, 2 out]
            n247 = RT FIFO Write(0:w506, 1:w505, 3:w503) -> (8:w504:refnum<k33>, 11:w502:errorcluster)  [unwired: 2 in, 2 out]
          }
        }
        n248 = call "FPGA Write.vi"("FPGA VI Reference IN"=w468, "Laser Signal Timing IN"=w493, "ephys_clock_timing IN"=w473, "frame_clock_timing IN"=w472, "Triggers IN"=w487, "Water Valve ON Time IN"=w494, "Error IN"=w477, "Analog Outputs IN"=w480) -> ("FPGA VI Reference OUT"=w475:refnum<k20>, "Error OUT"=w476:errorcluster)  [unwired: 6 in]
        n249 = node-c288() -> ()  [unwired: 1 in, 1 out]
      }
      n250 = while {
        stop <- FALSE stop-if-true
        (unwired) TRUE ("want seconds? (F)")
        # "Functional Global waiting\nfor Start Test shared variable\nto change state."
        # "Update Loop (Low Priority)"
        n251 = local read "Time into Trial"() -> (w72:dbl)
        n252 = shared-variable "RT CompactRIO Target\\Shared Variables.lvlib\\Timeout Timer"() -> (→"Timeout Timer":dbl)  [unwired: 1 in, 1 out]
        n253 = shared-variable "RT CompactRIO Target\\Shared Variables.lvlib\\Timeout?"() -> (→"Timeout?":bool)  [unwired: 1 in, 1 out]
        n254 = local read "Trial Fraction"() -> (w65:dbl)
        n255 = shared-variable "RT CompactRIO Target\\Shared Variables.lvlib\\Trial Distances"() -> (w68:dbl[])  [unwired: 1 in, 1 out]
        n256 = shared-variable "RT CompactRIO Target\\Shared Variables.lvlib\\Time Into Trial"(w72) -> ()  [unwired: 1 in, 1 out]
        n257 = Get Date/Time String() -> (date string=w78:string, time string=w77:string)  [unwired: 3 in]
        "cRIO System Time" <- w77
        "cRIO System Date" <- w78
        n258 = shared-variable "RT CompactRIO Target\\Shared Variables.lvlib\\Trial Fraction"(w65) -> ()  [unwired: 1 in, 1 out]
        n259 = Index Array(array=w68) -> (element #1=→"cur_trial_distance":dbl, element #2=w66:dbl)  [unwired: 2 in]
        n260 = Build Array(w78, w77) -> (w76:string[])
        n261 = shared-variable "RT CompactRIO Target\\Shared Variables.lvlib\\cRIO System DateTime"(w76) -> ()  [unwired: 1 in, 1 out]
        n262 = shared-variable "RT CompactRIO Target\\Shared Variables.lvlib\\Start Test"() -> (w64:bool)  [unwired: 1 in, 1 out]
        "Start Test" <- w64
        n263 = local read "Trial Running Graph Flag"() -> (w63:bool)
        n264 = while {
          shift-right: [w131] -> _
          shift-left: _ -> [w133]
          tunnel: w64 -> [w131]
          tunnel: [w132] -> w73
          tunnel: [w131] -> w74
          stop <- TRUE stop-if-true
          n265 = Not Equal?(x=w133, y=w131) -> (x != y?=w132:bool)
        }
        n266 = case shown="True" w73 {
          tunnel: w74 -> [_ w116]
          frame False {
          }
          frame True {
            n267 = case shown="False" w116 {
              frame False {
                n268 = stacked-sequence {
                  frame #0 {
                    n269 = Obtain Queue(name (unnamed)="RT", element data type=Control_RT_Code."Initialize" ("Command RT Code")) -> (queue out=w120:refnum<queue>, error out=w121:errorcluster)  [unwired: 3 in, 1 out]
                    n270 = Enqueue Element(queue=w120, element=Control_RT_Code."Stop Trial", error in (no error)=w121) -> ()  [unwired: 1 in, 3 out]
                  }
                  frame #1 {
                    n271 = Obtain Queue(name (unnamed)="Stats", element data type=cluster{"Numeric":dbl, "Numeric":dbl}[] [] ("array of clusters")) -> (queue out=w124:refnum<queue>, error out=w125:errorcluster)  [unwired: 3 in, 1 out]
                    n272 = Flush Queue(queue=w124, error in (no error)=w125) -> ()  [unwired: 3 out]
                  }
                }
              }
              frame True {
                n273 = Obtain Queue(name (unnamed)="RT", element data type=Control_RT_Code."Initialize" ("Command RT Code")) -> (queue out=w128:refnum<queue>, error out=w129:errorcluster)  [unwired: 3 in, 1 out]
                n274 = Enqueue Element(queue=w128, element=Control_RT_Code."Start New Test", error in (no error)=w129) -> ()  [unwired: 1 in, 3 out]
              }
            }
          }
        }
        n275 = while {
          tunnel: w66 -> [w87]
          tunnel: w65 -> [w86]
          tunnel: w63 -> [w85]
          tunnel: w64 -> [w80]
          shift-right: [w84] -> _
          shift-left: _ -> [w83]
          shift-right: [w82] -> _
          shift-left: _ -> [w81]
          stop <- TRUE stop-if-true
          # "For Lateral Distance History Graph and Histogram"
          n276 = case shown="False" w85 {
            tunnel: w87 -> [_ w105]
            tunnel: w86 -> [_ w111]
            tunnel: w81 -> [w91 w110]
            tunnel: [w93 w108] -> w84
            tunnel: w83 -> [w92 w109]
            tunnel: [w93 w107] -> w82
            tunnel: w80 -> [w88 _]
            frame False {
              w93 = dbl[] []
              n277 = local read "Flag - Lat Dist History"() -> (w89:bool)
              n278 = And(x=w89, y=w88) -> (x .and. y?=w90:bool)
              n279 = case shown="True" w90 {
                tunnel: w92 -> [_ w95]
                tunnel: w91 -> [_ w94]
                frame False {
                }
                frame True {
                  n280 = stacked-sequence {
                    tunnel: w95 -> [w96 _]
                    tunnel: w94 -> [w97 _]
                    frame #0 {
                      n281 = Build Cluster Array ("Index & Bundle Cluster Array")(w97, w96) -> (w98:cluster{"Trial Fraction":dbl, "Numeric":dbl}[])
                      n282 = Obtain Queue(name (unnamed)="Stats", element data type=cluster{"Numeric":dbl, "Numeric":dbl}[] [] ("array of clusters")) -> (queue out=w101:refnum<queue>, error out=w100:errorcluster)  [unwired: 3 in, 1 out]
                      n283 = Enqueue Element(queue=w101, element=w98, error in (no error)=w100) -> ()  [unwired: 1 in, 3 out]
                    }
                    frame #1 {
                      n284 = local write "Trial Running Graph Flag"(TRUE ("Trial Running Graph Flag")) -> ()
                      n285 = local write "Flag - Lat Dist History"(FALSE ("Flag - Update Lateral Dist History")) -> ()
                    }
                  }
                }
              }
            }
            frame True {
              n286 = disable-structure shown="Enabled" {
                disable-tunnel: [w112 w115] -> w106
                disable-tunnel: w105 -> [_ w115]
                frame Disabled {
                  n287 = Random Number (0-1)() -> (number: 0 to 1=w114:dbl)
                  n288 = Multiply(x=w114, y=20.0) -> (x*y=w112:dbl)
                }
                frame Enabled {
                }
              }
              n289 = Build Array (concatenate)(w109, w106) -> (w108:dbl[])
              n290 = Build Array (concatenate)(w110, w111) -> (w107:dbl[])
            }
          }
        }
        n291 = Wait (ms)(milliseconds to wait=u32 30) -> ()  [unwired: 1 out]
      }
      n292 = while {
        tunnel: w26 -> [w142]
        tunnel: w25 -> [w141]
        tunnel: [w140] -> w28
        tunnel: [w139] -> w27
        i -> [w135]
        stop <- FALSE stop-if-true
        n293 = Dequeue Element(queue=w142, timeout in ms (-1)=-1, error in (no error)=w141) -> (queue out=w140:refnum<queue>, element=w137:cluster{"Numeric":dbl, "Numeric":dbl}[], error out=w139:errorcluster)  [unwired: 1 out]
        n294 = call "Lateral Distance History.vi"("array of clusters"=w137, "Trial Index"=w135) -> ("Lateral Trial History"=→"Lateral Trial History":dbl[][])  [unwired: 9 in]
        "Numeric" <- w135
      }
      n295 = Release Queue(queue=w28, error in (no error)=w27) -> ()  [unwired: 1 in, 3 out]
      n296 = node-c288(w61) -> ()  [unwired: 1 out]
      n297 = RT FIFO Delete(0:w51, 3:w52) -> (11:w50:errorcluster)  [unwired: 1 in]
      n298 = RT FIFO Delete(0:w16, 3:w14) -> ()  [unwired: 1 in, 1 out]
      n299 = xnode "Close FPGA VI Reference"("FPGA VI Reference In"=w55, "error in"=w60) -> ("error out"=w54:errorcluster)
      n300 = Release Queue(queue=w34, error in (no error)=w33) -> (error out=w31:errorcluster)  [unwired: 1 in, 2 out]
    }
  }
  n301 = Merge Errors(w13, w12, w11, w10, w7, w8) -> (→"Error Out":errorcluster)
